vi "SelectRobotConfig.vi"(1 "Robot ID":T16) -> (0 "Selected Config":T1={"Motors"={"DriveLeftPrimary"={"CAN Address"=1, "Invert"=FALSE, "InvertSensor"=FALSE, "Unit Conversion Factor"=0.0, "Brake Mode"=enum."Override to Brake", "Reverse Limt Switch Mode"=enum."Normally Closed", "Forward Limt Swith Mode"=enum."Normally Closed"}, "DriveLeftSecondary1"={"CAN Address"=2, "Invert"=FALSE, "InvertSensor"=FALSE, "Unit Conversion Factor"=0.0, "Brake Mode"=enum."Override to Brake", "Reverse Limt Switch Mode"=enum."Normally Closed", "Forward Limt Swith Mode"=enum."Normally Closed"}, "DriveRightPrimary"={"CAN Address"=3, "Invert"=FALSE, "InvertSensor"=FALSE, "Unit Conversion Factor"=0.0, "Brake Mode"=enum."Override to Brake", "Reverse Limt Switch Mode"=enum."Normally Closed", "Forward Limt Swith Mode"=enum."Normally Closed"}, "DriveRightSecondary1"={"CAN Address"=4, "Invert"=FALSE, "InvertSensor"=FALSE, "Unit Conversion Factor"=0.0, "Brake Mode"=enum."Override to Brake", "Reverse Limt Switch Mode"=enum."Normally Closed", "Forward Limt Swith Mode"=enum."Normally Closed"}, "RightIntake"={"CAN Address"=8, "Invert"=FALSE, "InvertSensor"=FALSE, "Unit Conversion Factor"=0.0, "Brake Mode"=enum."Override to Brake", "Reverse Limt Switch Mode"=enum."Normally Closed", "Forward Limt Swith Mode"=enum."Normally Closed"}, "LeftIntake"={"CAN Address"=7, "Invert"=FALSE, "InvertSensor"=FALSE, "Unit Conversion Factor"=0.0, "Brake Mode"=enum."Override to Brake", "Reverse Limt Switch Mode"=enum."Normally Closed", "Forward Limt Swith Mode"=enum."Normally Closed"}, "ArmPivot"={"CAN Address"=5, "Invert"=FALSE, "InvertSensor"=FALSE, "Unit Conversion Factor"=0.0, "Brake Mode"=enum."Override to Brake", "Reverse Limt Switch Mode"=enum."Normally Closed", "Forward Limt Swith Mode"=enum."Normally Closed"}, "ArmExtend"={"CAN Address"=6, "Invert"=FALSE, "InvertSensor"=FALSE, "Unit Conversion Factor"=0.0, "Brake Mode"=enum."Override to Brake", "Reverse Limt Switch Mode"=enum."Normally Closed", "Forward Limt Swith Mode"=enum."Normally Closed"}, "ArmPivot2"={"CAN Address"=9, "Invert"=FALSE, "InvertSensor"=FALSE, "Unit Conversion Factor"=0.0, "Brake Mode"=enum."Override to Brake", "Reverse Limt Switch Mode"=enum."Normally Closed", "Forward Limt Swith Mode"=enum."Normally Closed"}, "Climber"={"CAN Address"=10, "Invert"=FALSE, "InvertSensor"=FALSE, "Unit Conversion Factor"=0.0, "Brake Mode"=enum."Override to Brake", "Reverse Limt Switch Mode"=enum."Disabled", "Forward Limt Swith Mode"=enum."Disabled"}, "CameraPole"={"CAN Address"=11, "Invert"=FALSE, "InvertSensor"=FALSE, "Unit Conversion Factor"=0.0, "Brake Mode"=enum."Override to Brake", "Reverse Limt Switch Mode"=enum."Disabled", "Forward Limt Swith Mode"=enum."Disabled"}}, "Sensors"={"IMU"={"Yaw Axis"=enum."Z", "SPI Bus"=enum."SPI MXP", "AHRS Algorithm"=enum."Complementary", "Calibration Time (s)"=3.0, "Calibrate On Open"=TRUE}, "LimitSwitch1"={"DIOChannel"=enum."DIO 0", "Active Low"=FALSE}, "LimitSwitch2"={"DIOChannel"=enum."DIO 1", "Active Low"=FALSE}, "BeamBreak"={"DIOChannel"=enum."DIO 2", "Active Low"=FALSE}, "JeVois"={"Baud Rate"=9600, "Parity"=0, "Data Bits"=8, "Stop Bits"=10, "Termination Char (0xA = '\\n' = LF)"=10, "Enable Termination Char? (T)"=TRUE, "Flow Control"=0, "Timeout Value (ms)"=5000, "Serial Port"=enum."Onboard RS-232"}}, "PID"={"ArmExtend"={"P"=0.0, "I"=0.0, "D"=0.0, "F"=0.0, "IZone"=0.0}, "ArmRotate"={"P"=0.0, "I"=0.0, "D"=0.0, "F"=0.0, "IZone"=0.0}, "Drive"={"P"=0.0, "I"=0.0, "D"=0.0, "F"=0.0, "IZone"=0.0}, "DriveGyro Kp ((in/sec)/deg)"=0.0, "CameraPole"={"P"=0.0, "I"=0.0, "D"=0.0, "F"=0.0, "IZone"=0.0}}, "Solenoids"={"ArmClaw"={"Forward Channel"=enum."Solenoid 0", "Invert"=FALSE, "Reverse Channel"=enum."Solenoid 0"}, "IntakeExtend"={"Forward Channel"=enum."Solenoid 1", "Invert"=FALSE, "Reverse Channel"=enum."Solenoid 0"}, "IntakeOpen"={"Forward Channel"=enum."Solenoid 2", "Invert"=FALSE, "Reverse Channel"=enum."Solenoid 0"}, " Shifter"={"Forward Channel"=enum."Solenoid 3", "Invert"=FALSE, "Reverse Channel"=enum."Solenoid 0"}}, "RobotDimensions "={"Length"=0.0, "Height"=0.0, "HeightOfBumpers"=0.0, "DistanceFromFrameEdgeToPyramid "=0.0, "HeightOfFrameToIntake"=0.0, "EdgeOfFrameToOrigin"=0.0}, "ArmHomePosition"={"Angle (rad)"=0.0, "Radius (in)"=0.0}, "CameraPoleHomeY (in)"=0.0, "CameraPoleCruiseVelocity"=0, "CameraPoleMaxAccel"=0} {"Sensors"."JeVois"."Flow Control" items=["None", "XON/XOFF", "RTS/CTS", "XON/XOFF & RTS/CTS", "DTR/DSR", "XON/XOFF & DTR/DSR"]; "Sensors"."JeVois"."Termination Char (0xA = '\\n' = LF)" format="%.0x"; "Sensors"."JeVois"."Stop Bits" items=["1.0"=10, "1.5"=15, "2.0"=20]; "Sensors"."JeVois"."Parity" items=["None", "Odd", "Even", "Mark", "Space"]})   [LabVIEW 2017]
uses:
  TypeDefs/RobotID.ctl
  TypeDefs/ConfigComponents/Config_Robot.ctl
  TypeDefs/ConfigComponents/Config_Motor.ctl
  <vilib>/Rock Robotics/WPI/ThirdParty/Phoenix-LabVIEW/Motor Controller/Controls/CTRE_Phoenix_MotorControl_NeutralMode.ctl
  <vilib>/Rock Robotics/WPI/ThirdParty/Phoenix-LabVIEW/Motor Controller/Controls/CTRE_Phoenix_MotorControl_LimitSwitchNormal.ctl
  TypeDefs/ConfigComponents/Config_IMU.ctl
  <vilib>/Rock Robotics/SystemInterfaces/spilib/spi_bus.ctl
  TypeDefs/ConfigComponents/Config_DigitalIO.ctl
  <vilib>/Rock Robotics/SystemInterfaces/DIO/FPGA_DIOChannel.ctl
  TypeDefs/ConfigComponents/Config_SerialPort.ctl
  <vilib>/Rock Robotics/WPI/SerialPort/WPI_SerialPort.ctl
  TypeDefs/ConfigComponents/Config_PIDParams.ctl
  TypeDefs/ConfigComponents/Config_DoubleSolenoid.ctl
  <vilib>/Rock Robotics/WPI/Solenoid/WPI_SolenoidChannel.ctl
  TypeDefs/ConfigComponents/Config_Dimensions.ctl
  TypeDefs/ConfigComponents/Config_ArmHome.ctl
panel:
  in  "Programming Robot":T1={"Motors"={"DriveLeftPrimary"={"CAN Address"=1, "Invert"=FALSE, "InvertSensor"=FALSE, "Unit Conversion Factor"=325.9493, "Brake Mode"=enum."Override to Brake", "Reverse Limt Switch Mode"=enum."Disabled", "Forward Limt Swith Mode"=enum."Disabled"}, "DriveLeftSecondary1"={"CAN Address"=2, "Invert"=FALSE, "InvertSensor"=FALSE, "Unit Conversion Factor"=0.0, "Brake Mode"=enum."Override to Brake", "Reverse Limt Switch Mode"=enum."Disabled", "Forward Limt Swith Mode"=enum."Disabled"}, "DriveRightPrimary"={"CAN Address"=3, "Invert"=FALSE, "InvertSensor"=FALSE, "Unit Conversion Factor"=325.9493, "Brake Mode"=enum."Override to Brake", "Reverse Limt Switch Mode"=enum."Disabled", "Forward Limt Swith Mode"=enum."Disabled"}, "DriveRightSecondary1"={"CAN Address"=4, "Invert"=FALSE, "InvertSensor"=FALSE, "Unit Conversion Factor"=0.0, "Brake Mode"=enum."Override to Brake", "Reverse Limt Switch Mode"=enum."Disabled", "Forward Limt Swith Mode"=enum."Disabled"}, "RightIntake"={"CAN Address"=8, "Invert"=TRUE, "InvertSensor"=FALSE, "Unit Conversion Factor"=0.0, "Brake Mode"=enum."Override to Brake", "Reverse Limt Switch Mode"=enum."Disabled", "Forward Limt Swith Mode"=enum."Disabled"}, "LeftIntake"={"CAN Address"=7, "Invert"=TRUE, "InvertSensor"=FALSE, "Unit Conversion Factor"=0.0, "Brake Mode"=enum."Override to Brake", "Reverse Limt Switch Mode"=enum."Disabled", "Forward Limt Swith Mode"=enum."Disabled"}, "ArmPivot"={"CAN Address"=5, "Invert"=TRUE, "InvertSensor"=FALSE, "Unit Conversion Factor"=2610.0, "Brake Mode"=enum."Override to Brake", "Reverse Limt Switch Mode"=enum."Disabled", "Forward Limt Swith Mode"=enum."Disabled"}, "ArmExtend"={"CAN Address"=6, "Invert"=FALSE, "InvertSensor"=TRUE, "Unit Conversion Factor"=745.86, "Brake Mode"=enum."Override to Brake", "Reverse Limt Switch Mode"=enum."Disabled", "Forward Limt Swith Mode"=enum."Disabled"}, "ArmPivot2"={"CAN Address"=9, "Invert"=FALSE, "InvertSensor"=FALSE, "Unit Conversion Factor"=0.0, "Brake Mode"=enum."Override to Brake", "Reverse Limt Switch Mode"=enum."Disabled", "Forward Limt Swith Mode"=enum."Disabled"}, "Climber"={"CAN Address"=10, "Invert"=FALSE, "InvertSensor"=FALSE, "Unit Conversion Factor"=0.0, "Brake Mode"=enum."Override to Brake", "Reverse Limt Switch Mode"=enum."Disabled", "Forward Limt Swith Mode"=enum."Disabled"}, "CameraPole"={"CAN Address"=11, "Invert"=FALSE, "InvertSensor"=FALSE, "Unit Conversion Factor"=0.0, "Brake Mode"=enum."Override to Brake", "Reverse Limt Switch Mode"=enum."Disabled", "Forward Limt Swith Mode"=enum."Disabled"}}, "Sensors"={"IMU"={"Yaw Axis"=enum."Z", "SPI Bus"=enum."SPI MXP", "AHRS Algorithm"=enum."Complementary", "Calibration Time (s)"=3.0, "Calibrate On Open"=TRUE}, "LimitSwitch1"={"DIOChannel"=enum."DIO 0", "Active Low"=FALSE}, "LimitSwitch2"={"DIOChannel"=enum."DIO 1", "Active Low"=FALSE}, "BeamBreak"={"DIOChannel"=enum."DIO 2", "Active Low"=FALSE}, "JeVois"={"Baud Rate"=9600, "Parity"=0, "Data Bits"=8, "Stop Bits"=10, "Termination Char (0xA = '\\n' = LF)"=10, "Enable Termination Char? (T)"=TRUE, "Flow Control"=0, "Timeout Value (ms)"=100, "Serial Port"=enum."USB 1"}}, "PID"={"ArmExtend"={"P"=0.3, "I"=0.0, "D"=0.0, "F"=0.02, "IZone"=0.0}, "ArmRotate"={"P"=1.7, "I"=0.0, "D"=0.0, "F"=0.25, "IZone"=0.0}, "Drive"={"P"=0.2, "I"=0.0025, "D"=0.0, "F"=0.22, "IZone"=2000.0}, "DriveGyro Kp ((in/sec)/deg)"=0.0, "CameraPole"={"P"=0.0, "I"=0.0, "D"=0.0, "F"=0.0, "IZone"=0.0}}, "Solenoids"={"ArmClaw"={"Forward Channel"=enum."Solenoid 1", "Invert"=FALSE, "Reverse Channel"=enum."Solenoid 6"}, "IntakeExtend"={"Forward Channel"=enum."Solenoid 2", "Invert"=FALSE, "Reverse Channel"=enum."Solenoid 5"}, "IntakeOpen"={"Forward Channel"=enum."Solenoid 3", "Invert"=FALSE, "Reverse Channel"=enum."Solenoid 4"}, " Shifter"={"Forward Channel"=enum."Solenoid 0", "Invert"=FALSE, "Reverse Channel"=enum."Solenoid 7"}}, "RobotDimensions "={"Length"=32.0, "Height"=50.0, "HeightOfBumpers"=6.0, "DistanceFromFrameEdgeToPyramid "=11.5, "HeightOfFrameToIntake"=0.0, "EdgeOfFrameToOrigin"=4.5}, "ArmHomePosition"={"Angle (rad)"=-0.4712, "Radius (in)"=-43.75}, "CameraPoleHomeY (in)"=0.0, "CameraPoleCruiseVelocity"=0, "CameraPoleMaxAccel"=0} {"Sensors"."JeVois"."Flow Control" items=["None", "XON/XOFF", "RTS/CTS", "XON/XOFF & RTS/CTS", "DTR/DSR", "XON/XOFF & DTR/DSR"]; "Sensors"."JeVois"."Termination Char (0xA = '\\n' = LF)" format="%.0x"; "Sensors"."JeVois"."Stop Bits" items=["1.0"=10, "1.5"=15, "2.0"=20]; "Sensors"."JeVois"."Parity" items=["None", "Odd", "Even", "Mark", "Space"]}
  in  "Practice Robot":T1={"Motors"={"DriveLeftPrimary"={"CAN Address"=1, "Invert"=FALSE, "InvertSensor"=FALSE, "Unit Conversion Factor"=327.6, "Brake Mode"=enum."Override to Brake", "Reverse Limt Switch Mode"=enum."Disabled", "Forward Limt Swith Mode"=enum."Disabled"}, "DriveLeftSecondary1"={"CAN Address"=2, "Invert"=FALSE, "InvertSensor"=FALSE, "Unit Conversion Factor"=0.0, "Brake Mode"=enum."Override to Brake", "Reverse Limt Switch Mode"=enum."Disabled", "Forward Limt Swith Mode"=enum."Disabled"}, "DriveRightPrimary"={"CAN Address"=3, "Invert"=FALSE, "InvertSensor"=FALSE, "Unit Conversion Factor"=323.76, "Brake Mode"=enum."Override to Brake", "Reverse Limt Switch Mode"=enum."Disabled", "Forward Limt Swith Mode"=enum."Disabled"}, "DriveRightSecondary1"={"CAN Address"=4, "Invert"=FALSE, "InvertSensor"=FALSE, "Unit Conversion Factor"=0.0, "Brake Mode"=enum."Override to Brake", "Reverse Limt Switch Mode"=enum."Disabled", "Forward Limt Swith Mode"=enum."Disabled"}, "RightIntake"={"CAN Address"=8, "Invert"=TRUE, "InvertSensor"=FALSE, "Unit Conversion Factor"=0.0, "Brake Mode"=enum."Override to Brake", "Reverse Limt Switch Mode"=enum."Disabled", "Forward Limt Swith Mode"=enum."Disabled"}, "LeftIntake"={"CAN Address"=7, "Invert"=TRUE, "InvertSensor"=FALSE, "Unit Conversion Factor"=0.0, "Brake Mode"=enum."Override to Brake", "Reverse Limt Switch Mode"=enum."Disabled", "Forward Limt Swith Mode"=enum."Disabled"}, "ArmPivot"={"CAN Address"=5, "Invert"=TRUE, "InvertSensor"=FALSE, "Unit Conversion Factor"=2610.0, "Brake Mode"=enum."Override to Brake", "Reverse Limt Switch Mode"=enum."Normally Closed", "Forward Limt Swith Mode"=enum."Disabled"}, "ArmExtend"={"CAN Address"=6, "Invert"=FALSE, "InvertSensor"=TRUE, "Unit Conversion Factor"=745.86, "Brake Mode"=enum."Override to Brake", "Reverse Limt Switch Mode"=enum."Normally Closed", "Forward Limt Swith Mode"=enum."Disabled"}, "ArmPivot2"={"CAN Address"=9, "Invert"=FALSE, "InvertSensor"=FALSE, "Unit Conversion Factor"=0.0, "Brake Mode"=enum."Override to Brake", "Reverse Limt Switch Mode"=enum."Disabled", "Forward Limt Swith Mode"=enum."Disabled"}, "Climber"={"CAN Address"=10, "Invert"=FALSE, "InvertSensor"=FALSE, "Unit Conversion Factor"=0.0, "Brake Mode"=enum."Override to Brake", "Reverse Limt Switch Mode"=enum."Disabled", "Forward Limt Swith Mode"=enum."Disabled"}, "CameraPole"={"CAN Address"=11, "Invert"=FALSE, "InvertSensor"=TRUE, "Unit Conversion Factor"=0.0, "Brake Mode"=enum."Override to Brake", "Reverse Limt Switch Mode"=enum."Disabled", "Forward Limt Swith Mode"=enum."Disabled"}}, "Sensors"={"IMU"={"Yaw Axis"=enum."Z", "SPI Bus"=enum."SPI MXP", "AHRS Algorithm"=enum."Complementary", "Calibration Time (s)"=3.0, "Calibrate On Open"=TRUE}, "LimitSwitch1"={"DIOChannel"=enum."DIO 0", "Active Low"=FALSE}, "LimitSwitch2"={"DIOChannel"=enum."DIO 1", "Active Low"=FALSE}, "BeamBreak"={"DIOChannel"=enum."DIO 2", "Active Low"=FALSE}, "JeVois"={"Baud Rate"=9600, "Parity"=0, "Data Bits"=8, "Stop Bits"=10, "Termination Char (0xA = '\\n' = LF)"=10, "Enable Termination Char? (T)"=TRUE, "Flow Control"=0, "Timeout Value (ms)"=100, "Serial Port"=enum."USB 1"}}, "PID"={"ArmExtend"={"P"=0.3, "I"=0.0, "D"=0.0, "F"=0.02, "IZone"=0.0}, "ArmRotate"={"P"=1.7, "I"=0.0, "D"=0.0, "F"=0.25, "IZone"=0.0}, "Drive"={"P"=0.4, "I"=0.0015, "D"=0.0, "F"=0.35, "IZone"=1000.0}, "DriveGyro Kp ((in/sec)/deg)"=0.0, "CameraPole"={"P"=0.0, "I"=0.0, "D"=0.0, "F"=0.0, "IZone"=0.0}}, "Solenoids"={"ArmClaw"={"Forward Channel"=enum."Solenoid 1", "Invert"=FALSE, "Reverse Channel"=enum."Solenoid 6"}, "IntakeExtend"={"Forward Channel"=enum."Solenoid 2", "Invert"=FALSE, "Reverse Channel"=enum."Solenoid 5"}, "IntakeOpen"={"Forward Channel"=enum."Solenoid 3", "Invert"=FALSE, "Reverse Channel"=enum."Solenoid 4"}, " Shifter"={"Forward Channel"=enum."Solenoid 0", "Invert"=FALSE, "Reverse Channel"=enum."Solenoid 7"}}, "RobotDimensions "={"Length"=32.0, "Height"=50.0, "HeightOfBumpers"=6.0, "DistanceFromFrameEdgeToPyramid "=11.5, "HeightOfFrameToIntake"=0.0, "EdgeOfFrameToOrigin"=4.5}, "ArmHomePosition"={"Angle (rad)"=-0.4712, "Radius (in)"=-43.75}, "CameraPoleHomeY (in)"=0.0, "CameraPoleCruiseVelocity"=0, "CameraPoleMaxAccel"=0} {"Sensors"."JeVois"."Flow Control" items=["None", "XON/XOFF", "RTS/CTS", "XON/XOFF & RTS/CTS", "DTR/DSR", "XON/XOFF & DTR/DSR"]; "Sensors"."JeVois"."Termination Char (0xA = '\\n' = LF)" format="%.0x"; "Sensors"."JeVois"."Stop Bits" items=["1.0"=10, "1.5"=15, "2.0"=20]; "Sensors"."JeVois"."Parity" items=["None", "Odd", "Even", "Mark", "Space"]}
  in  "Competition Robot":T1={"Motors"={"DriveLeftPrimary"={"CAN Address"=1, "Invert"=FALSE, "InvertSensor"=FALSE, "Unit Conversion Factor"=322.044, "Brake Mode"=enum."Override to Brake", "Reverse Limt Switch Mode"=enum."Disabled", "Forward Limt Swith Mode"=enum."Disabled"}, "DriveLeftSecondary1"={"CAN Address"=2, "Invert"=FALSE, "InvertSensor"=FALSE, "Unit Conversion Factor"=0.0, "Brake Mode"=enum."Override to Brake", "Reverse Limt Switch Mode"=enum."Disabled", "Forward Limt Swith Mode"=enum."Disabled"}, "DriveRightPrimary"={"CAN Address"=3, "Invert"=FALSE, "InvertSensor"=FALSE, "Unit Conversion Factor"=322.044, "Brake Mode"=enum."Override to Brake", "Reverse Limt Switch Mode"=enum."Disabled", "Forward Limt Swith Mode"=enum."Disabled"}, "DriveRightSecondary1"={"CAN Address"=4, "Invert"=FALSE, "InvertSensor"=FALSE, "Unit Conversion Factor"=0.0, "Brake Mode"=enum."Override to Brake", "Reverse Limt Switch Mode"=enum."Disabled", "Forward Limt Swith Mode"=enum."Disabled"}, "RightIntake"={"CAN Address"=8, "Invert"=TRUE, "InvertSensor"=FALSE, "Unit Conversion Factor"=0.0, "Brake Mode"=enum."Override to Brake", "Reverse Limt Switch Mode"=enum."Disabled", "Forward Limt Swith Mode"=enum."Disabled"}, "LeftIntake"={"CAN Address"=7, "Invert"=TRUE, "InvertSensor"=FALSE, "Unit Conversion Factor"=0.0, "Brake Mode"=enum."Override to Brake", "Reverse Limt Switch Mode"=enum."Disabled", "Forward Limt Swith Mode"=enum."Disabled"}, "ArmPivot"={"CAN Address"=5, "Invert"=TRUE, "InvertSensor"=FALSE, "Unit Conversion Factor"=2610.0, "Brake Mode"=enum."Override to Brake", "Reverse Limt Switch Mode"=enum."Disabled", "Forward Limt Swith Mode"=enum."Disabled"}, "ArmExtend"={"CAN Address"=6, "Invert"=FALSE, "InvertSensor"=TRUE, "Unit Conversion Factor"=745.86, "Brake Mode"=enum."Override to Brake", "Reverse Limt Switch Mode"=enum."Normally Closed", "Forward Limt Swith Mode"=enum."Disabled"}, "ArmPivot2"={"CAN Address"=9, "Invert"=FALSE, "InvertSensor"=FALSE, "Unit Conversion Factor"=0.0, "Brake Mode"=enum."Override to Brake", "Reverse Limt Switch Mode"=enum."Disabled", "Forward Limt Swith Mode"=enum."Disabled"}, "Climber"={"CAN Address"=10, "Invert"=FALSE, "InvertSensor"=FALSE, "Unit Conversion Factor"=0.0, "Brake Mode"=enum."Override to Brake", "Reverse Limt Switch Mode"=enum."Disabled", "Forward Limt Swith Mode"=enum."Disabled"}, "CameraPole"={"CAN Address"=11, "Invert"=FALSE, "InvertSensor"=TRUE, "Unit Conversion Factor"=0.0, "Brake Mode"=enum."Override to Brake", "Reverse Limt Switch Mode"=enum."Disabled", "Forward Limt Swith Mode"=enum."Disabled"}}, "Sensors"={"IMU"={"Yaw Axis"=enum."Z", "SPI Bus"=enum."SPI MXP", "AHRS Algorithm"=enum."Complementary", "Calibration Time (s)"=3.0, "Calibrate On Open"=TRUE}, "LimitSwitch1"={"DIOChannel"=enum."DIO 0", "Active Low"=FALSE}, "LimitSwitch2"={"DIOChannel"=enum."DIO 1", "Active Low"=FALSE}, "BeamBreak"={"DIOChannel"=enum."DIO 2", "Active Low"=FALSE}, "JeVois"={"Baud Rate"=9600, "Parity"=0, "Data Bits"=8, "Stop Bits"=10, "Termination Char (0xA = '\\n' = LF)"=10, "Enable Termination Char? (T)"=TRUE, "Flow Control"=0, "Timeout Value (ms)"=100, "Serial Port"=enum."USB 1"}}, "PID"={"ArmExtend"={"P"=0.3, "I"=0.0, "D"=0.0, "F"=0.02, "IZone"=0.0}, "ArmRotate"={"P"=1.7, "I"=0.0, "D"=0.0, "F"=0.25, "IZone"=0.0}, "Drive"={"P"=0.4, "I"=0.0015, "D"=0.0, "F"=0.35, "IZone"=1000.0}, "DriveGyro Kp ((in/sec)/deg)"=0.0, "CameraPole"={"P"=0.0, "I"=0.0, "D"=0.0, "F"=0.0, "IZone"=0.0}}, "Solenoids"={"ArmClaw"={"Forward Channel"=enum."Solenoid 1", "Invert"=FALSE, "Reverse Channel"=enum."Solenoid 6"}, "IntakeExtend"={"Forward Channel"=enum."Solenoid 2", "Invert"=FALSE, "Reverse Channel"=enum."Solenoid 5"}, "IntakeOpen"={"Forward Channel"=enum."Solenoid 3", "Invert"=FALSE, "Reverse Channel"=enum."Solenoid 4"}, " Shifter"={"Forward Channel"=enum."Solenoid 0", "Invert"=FALSE, "Reverse Channel"=enum."Solenoid 7"}}, "RobotDimensions "={"Length"=32.0, "Height"=50.0, "HeightOfBumpers"=6.0, "DistanceFromFrameEdgeToPyramid "=11.5, "HeightOfFrameToIntake"=0.0, "EdgeOfFrameToOrigin"=4.5}, "ArmHomePosition"={"Angle (rad)"=-0.4712, "Radius (in)"=-43.75}, "CameraPoleHomeY (in)"=0.0, "CameraPoleCruiseVelocity"=0, "CameraPoleMaxAccel"=0} {"Sensors"."JeVois"."Flow Control" items=["None", "XON/XOFF", "RTS/CTS", "XON/XOFF & RTS/CTS", "DTR/DSR", "XON/XOFF & DTR/DSR"]; "Sensors"."JeVois"."Termination Char (0xA = '\\n' = LF)" format="%.0x"; "Sensors"."JeVois"."Stop Bits" items=["1.0"=10, "1.5"=15, "2.0"=20]; "Sensors"."JeVois"."Parity" items=["None", "Odd", "Even", "Mark", "Space"]}
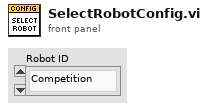
[diagram p1: front panel]
types:
  T1 = typedef "Config_Robot.ctl" = cluster{"Motors":cluster{"DriveLeftPrimary":T2, "DriveLeftSecondary1":T2, "DriveRightPrimary":T2, "DriveRightSecondary1":T2, "RightIntake":T2, "LeftIntake":T2, "ArmPivot":T2, "ArmExtend":T2, "ArmPivot2":T2, "Climber":T2, "CameraPole":T2}, "Sensors":cluster{"IMU":T5, "LimitSwitch1":T7, "LimitSwitch2":T7, "BeamBreak":T7, "JeVois":T9}, "PID":cluster{"ArmExtend":T11, "ArmRotate":T11, "Drive":T11, "DriveGyro Kp ((in/sec)/deg)":dbl, "CameraPole":T11}, "Solenoids":cluster{"ArmClaw":T12, "IntakeExtend":T12, "IntakeOpen":T12, " Shifter":T12}, "RobotDimensions ":T14, "ArmHomePosition":T15, "CameraPoleHomeY (in)":dbl, "CameraPoleCruiseVelocity":i32, "CameraPoleMaxAccel":i32}
  T2 = typedef "Config_Motor.ctl" = cluster{"CAN Address":u8, "Invert":bool, "InvertSensor":bool, "Unit Conversion Factor":dbl, "Brake Mode":T3, "Reverse Limt Switch Mode":T4, "Forward Limt Swith Mode":T4}
  T3 = typedef "CTRE_Phoenix_MotorControl_NeutralMode.ctl" = enum8{"EEPROMSetting", "Override to Coast", "Override to Brake"}
  T4 = typedef "CTRE_Phoenix_MotorControl_LimitSwitchNormal.ctl" = enum16{"Normally Open", "Normally Closed", "Disabled"}
  T5 = typedef "Config_IMU.ctl" = cluster{"Yaw Axis":enum16{"X", "Y", "Z"}, "SPI Bus":T6, "AHRS Algorithm":enum16{"Complementary", "Madgwick"}, "Calibration Time (s)":dbl, "Calibrate On Open":bool}
  T6 = typedef "spi_bus.ctl" = enum16{"SPI On-Board, CS0", "SPI On-Board, CS1", "SPI On-Board, CS2", "SPI On-Board, CS3", "SPI MXP", "Invalid"}
  T7 = typedef "Config_DigitalIO.ctl" = cluster{"DIOChannel":T8, "Active Low":bool}
  T8 = typedef "FPGA_DIOChannel.ctl" = enum8{"DIO 0", "DIO 1", "DIO 2", "DIO 3", "DIO 4", "DIO 5", "DIO 6", "DIO 7", "DIO 8", "DIO 9", "DIO MXP 0", "DIO MXP 1", "DIO MXP 2", "DIO MXP 3", "DIO MXP 4", "DIO MXP 5", "DIO MXP 6", "DIO MXP 7", "DIO MXP 8", "DIO MXP 9", "DIO MXP 10", "DIO MXP 11", "DIO MXP 12", "DIO MXP 13", "DIO MXP 14", "DIO MXP 15", "SPI Port CS1", "SPI Port CS2", "SPI Port CS3", "SPI Port MISO", "SPI Port MOSI", "Invalid"}
  T9 = typedef "Config_SerialPort.ctl" = cluster{"Baud Rate":u32, "Parity":u16, "Data Bits":u16, "Stop Bits":u16, "Termination Char (0xA = '\\n' = LF)":u8, "Enable Termination Char? (T)":bool, "Flow Control":u16, "Timeout Value (ms)":u32, "Serial Port":T10}
  T10 = typedef "WPI_SerialPort.ctl" = enum16{"Onboard RS-232", "MXP TTL", "USB 1", "USB 2"}
  T11 = typedef "Config_PIDParams.ctl" = cluster{"P":dbl, "I":dbl, "D":dbl, "F":dbl, "IZone":dbl}
  T12 = typedef "Config_DoubleSolenoid.ctl" = cluster{"Forward Channel":T13, "Invert":bool, "Reverse Channel":T13}
  T13 = typedef "WPI_SolenoidChannel.ctl" = enum8{"Solenoid 0", "Solenoid 1", "Solenoid 2", "Solenoid 3", "Solenoid 4", "Solenoid 5", "Solenoid 6", "Solenoid 7", "Invalid"}
  T14 = typedef "Config_Dimensions.ctl" = cluster{"Length":dbl, "Height":dbl, "HeightOfBumpers":dbl, "DistanceFromFrameEdgeToPyramid ":dbl, "HeightOfFrameToIntake":dbl, "EdgeOfFrameToOrigin":dbl}
  T15 = typedef "Config_ArmHome.ctl" = cluster{"Angle (rad)":dbl, "Radius (in)":dbl}
  T16 = typedef "RobotID.ctl" = enum16{"Competition", "Practice", "Programming"}
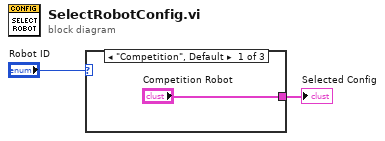
[diagram p0: block diagram]
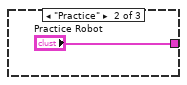
[diagram p2: hidden frame]
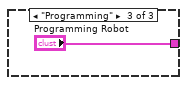
[diagram p3: hidden frame]
diagram:
  n1 = case shown="\"Competition\", Default" "Robot ID" {
    tunnel: ["Competition Robot" "Practice Robot" "Programming Robot"] -> w1
    frame "Competition", Default {
    }
    frame "Practice" {
    }
    frame "Programming" {
    }
  }
  "Selected Config" <- w1
